vi "Open Hardware.vi"(8 "error in (no error)":errorcluster, 11 "Instrument.FrameworkTemplate":refnum<class "Temperhum.Thorlabs.lvclass">) -> (0 "error out":errorcluster, 3 "Instrument.FrameworkTemplate out":refnum<class "Temperhum.Thorlabs.lvclass">)   [LabVIEW 2019, in "Temperhum.Thorlabs.lvclass"]
uses:
  Temperhum.Thorlabs.lvclass
  Typedefs/Thorlabs Type --enum.ctl
  Temperhum.Thorlabs.lvclass/Temperhum.Thorlabs.ctl
  Instrument.Temperhum/Instrument.Temperhum.lvclass
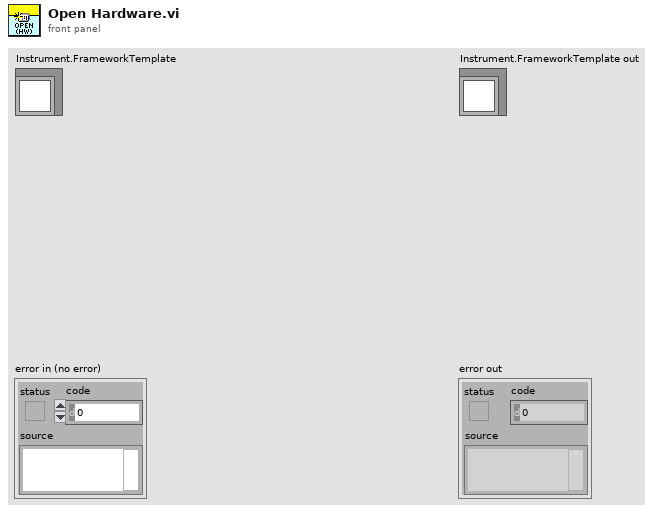
[diagram p1: front panel]
types:
  T1 = typedef "Temperhum.Thorlabs.lvclass/Thorlabs Type --enum.ctl" = enum16{"A", "B"}
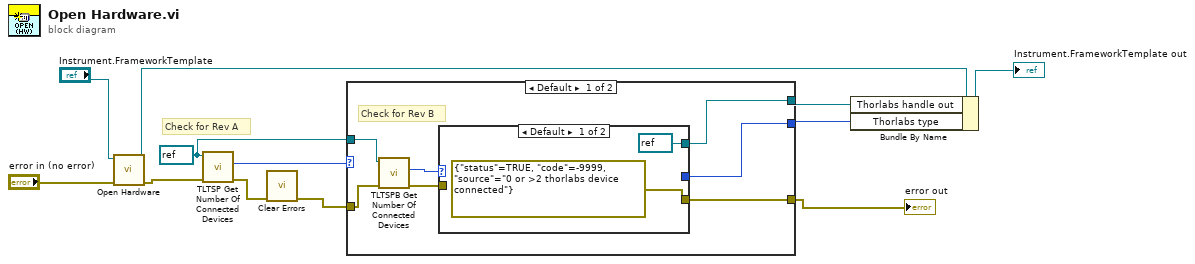
[diagram p0: block diagram]
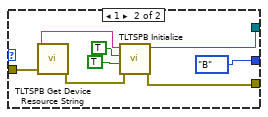
[diagram p2: hidden frame]
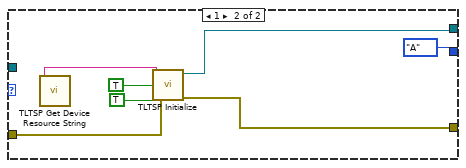
[diagram p3: hidden frame]
diagram:
  w6 = refnum<visa-resource-name> refnum ("instrument handle")
  # "Check for Rev A"
  n1 = call-parent "Open Hardware.vi"("error in (no error)"="error in (no error)", "Instrument.FrameworkTemplate"="Instrument.FrameworkTemplate") -> ("error out"=w4:errorcluster, "Instrument.FrameworkTemplate out"=w10:refnum<class "Temperhum.Thorlabs.lvclass">)  [unwired: 8 in]
  n2 = call <instrlib>:"TLTSP Get Number Of Connected Devices.vi"("error in (no error)"=w4, "instrument handle"=w6) -> ("error out"=w3:errorcluster, "Device Count"=w9:u32)  [unwired: 7 in, 1 out]
  n3 = call <vilib>:"Clear Errors.vi"("error in (no error)"=w3) -> ("error out"=w2:errorcluster)  [unwired: 5 in, 1 out]
  n4 = case shown="Default" w9 {
    tunnel: w2 -> [w19 w36]
    tunnel: [w14 w33] -> w8
    tunnel: [w16 w32] -> w7
    tunnel: w6 -> [w18 _]
    tunnel: [w13 Thorlabs_Type_--enum."A"] -> w5
    frame Default {
      # "Check for Rev B"
      n5 = call <instrlib>:"TLTSPB Get Number Of Connected Devices.vi"("error in (no error)"=w19, "instrument handle"=w18) -> ("error out"=w15:errorcluster, "Device Count"=w17:u32)  [unwired: 7 in, 1 out]
      n6 = case shown="Default" w17 {
        tunnel: [refnum<visa-resource-name> refnum ("instrument handle out") w28] -> w16
        tunnel: w15 -> [_ w27]
        tunnel: [errorcluster {"status"=TRUE, "code"=-9999, "source"="0 or >2 thorlabs device connected"} ("error out") w25] -> w14
        tunnel: [_ Thorlabs_Type_--enum."B"] -> w13
        frame Default {
        }
        frame 1 {
          n7 = call <instrlib>:"TLTSPB Get Device Resource String.vi"("error in (no error)"=w27) -> ("error out"=w26:errorcluster, "Resource Name"=w29:string)  [unwired: 8 in, 1 out]
          n8 = call <instrlib>:"TLTSPB Initialize.vi"("error in (no error)"=w26, "Reset Device (Reset Device)"=TRUE, "ID Query (Do Query)"=TRUE, "resource name"=w29) -> ("error out"=w25:errorcluster, "instrument handle out"=w28:refnum<visa-resource-name>)  [unwired: 6 in]
        }
      }
    }
    frame 1 {
      n9 = call <instrlib>:"TLTSP Get Device Resource String.vi"() -> ("Resource Name"=w31:string)  [unwired: 9 in, 2 out]
      n10 = call <instrlib>:"TLTSP Initialize.vi"("error in (no error)"=w36, "Reset Device (Reset Device)"=TRUE, "ID Query (Do Query)"=TRUE, "resource name"=w31) -> ("error out"=w33:errorcluster, "instrument handle out"=w32:refnum<visa-resource-name>)  [unwired: 6 in]
    }
  }
  "error out" <- w8
  n11 = Bundle By Name(cluster=w10, "Thorlabs handle out"=w7, "Thorlabs type"=w5) -> (→"Instrument.FrameworkTemplate out":refnum<class "Temperhum.Thorlabs.lvclass">)
